vi "ROI group-Average.vi"(9 "Data in":T4) -> (1 "ROI group data":T1, 3 "Averaged":bool)   [LabVIEW 2013]
uses:
  xcontrol/Interface VIs/Interface typedefs/Interface-Data array.ctl
  xcontrol/Interface VIs/Interface typedefs/Interface-Data format definition.ctl
  xcontrol/Typedefs/Xctl-XY data type definition.ctl
  xcontrol/Typedefs/Xctrl-ROI type enum.ctl
  <vilib>/Analysis/baseanly.llb/Mean (DBL).vi
  <vilib>/Analysis/NI_AALBase.lvlib
  xcontrol/XGrapher.xctl
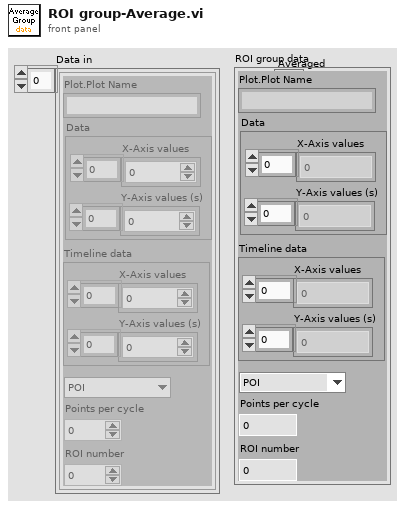
[diagram p1: front panel]
types:
  T1 = typedef "Interface-Data format definition.ctl" = cluster{"Plot.Plot Name":string, "Data":T2, "Timeline data":T2, "Type":T3, "Points per cycle":u16, "ROI number":u16}
  T2 = typedef "XGrapher.xctl/Xctl-XY data type definition.ctl" = cluster{"X-Axis values":sgl[], "Y-Axis values (s)":i32[]}
  T3 = typedef "Xctrl-ROI type enum.ctl" = enum16{"POI", "Mini-scan", "Group"}
  T4 = typedef "Interface-Data array.ctl" = T1[]
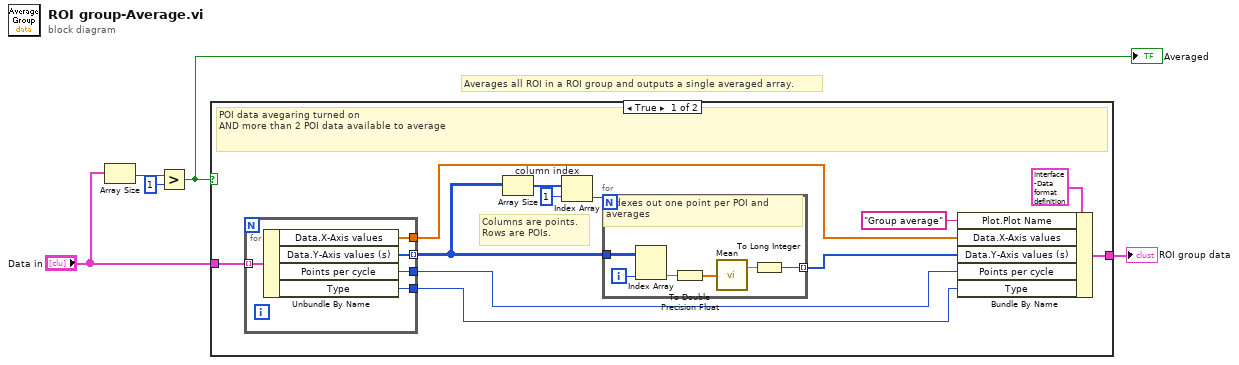
[diagram p0: block diagram]
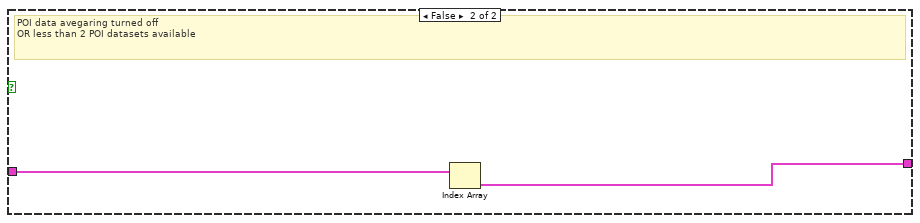
[diagram p2: hidden frame]
diagram:
  # "Averages all ROI in a ROI group and outputs a single averaged array."
  n1 = Array Size(array="Data in") -> (size(s)=w4:i32)
  n2 = Greater?(x=w4, y=1) -> (0:w5:bool)
  "Averaged" <- w5
  n3 = case shown="True" w5 {
    tunnel: "Data in" -> [w17 w30]
    tunnel: [w9 w29] -> w1
    frame True {
      w15 = 1  # column index
      # "Columns are points.\nRows are POIs."
      # "POI data avegaring turned on\nAND more than 2 POI data available to average"
      n4 = for {
        tunnel: w17 -> [w22] mode=indexing
        tunnel: [w21] -> w8 mode=indexing
        tunnel: [w20] -> w12
        tunnel: [w19] -> w13
        tunnel: [w18] -> w10
        n5 = Unbundle By Name(w22) -> ("Data.X-Axis values"=w19:sgl[], "Data.Y-Axis values (s)"=w21:i32[], "Points per cycle"=w20:u16, "Type"=w18:T3)
      }
      n6 = Array Size(array=w8) -> (size(s)=w16:i32[])
      n7 = Index Array(array=w16, index=w15) -> (element=w14:i32)
      n8 = for {
        N: w14 -> [_]
        tunnel: w8 -> [w27]
        tunnel: [w23] -> w7 mode=indexing
        i -> [w28]
        # "Indexes out one point per POI and averages"
        n9 = Index Array(array=w27, index (col)=w28) -> (element=w25:i32[])  [unwired: 1 in]
        n10 = To Double Precision Float(number=w25) -> (double precision float=w24:dbl[])
        n11 = call-poly <vilib>:"Mean.vi"("X"=w24) -> ("mean"=w26:dbl)  [unwired: 1 out]
        n12 = To Long Integer(number=w26) -> (32bit integer=w23:i32)
      }
      n13 = Bundle By Name(cluster=T1 {"Plot.Plot Name"="", "Data"={"X-Axis values"=[], "Y-Axis values (s)"=[]}, "Timeline data"={"X-Axis values"=[], "Y-Axis values (s)"=[]}, "Type"=enum."POI", "Points per cycle"=0, "ROI number"=0}, "Plot.Plot Name"="Group average", "Data.X-Axis values"=w13, "Data.Y-Axis values (s)"=w7, "Points per cycle"=w12, "Type"=w10) -> (w9:T1)
    }
    frame False {
      # "POI data avegaring turned off\nOR less than 2 POI datasets available"
      n14 = Index Array(array=w30) -> (element=w29:T1)  [unwired: 1 in]
    }
  }
  "ROI group data" <- w1
